vi "Configure Digitize Function.vi"(6 "Sample Rate (1E+6)":dbl=1000000.0, 7 "Manual Range (0)":dbl=1.0, 8 "error in (no error)":errorcluster, 9 "Count (1)":u32=1, 10 "Function":u16(ring) items=["Digitize Voltage", "Digitize Current"], 11 "VISA resource name":refnum<visa-resource-name>) -> (0 "error out":errorcluster, 3 "VISA resource name out":refnum<visa-resource-name>)   [LabVIEW 2025, in "Keithley DMM7510.lvlib"]
doc: "This VI selects which type of digitize function is active."
uses:
  Keithley DMM7510.lvlib
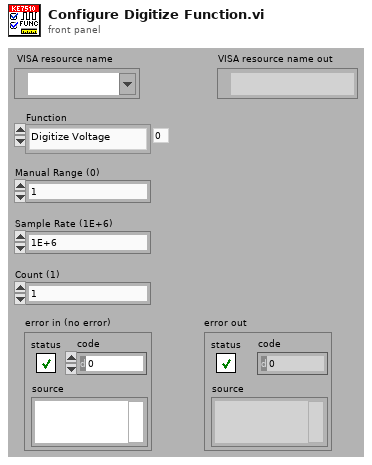
[diagram p1: front panel]
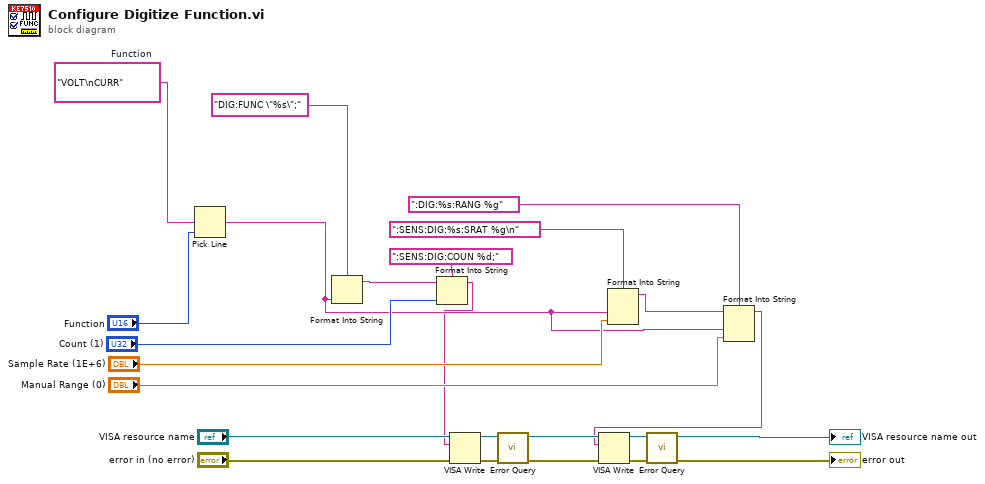
[diagram p0: block diagram]
diagram:
  w19 = "VOLT\nCURR"  # Function
  n1 = Pick Line(multi-line string=w19, line index="Function") -> (output string=w12:string)  [unwired: 1 out]
  n2 = Format Into String(format string="DIG:FUNC \"%s\";", w12) -> (resulting string=w10:string)  [unwired: 2 in, 1 out]
  n3 = Format Into String(format string=":SENS:DIG:COUN %d;", initial string=w10, "Count (1)") -> (resulting string=w9:string)  [unwired: 1 in, 1 out]
  n4 = VISA Write(VISA resource name="VISA resource name", write buffer=w9, error in (no error)="error in (no error)") -> (VISA resource name out=w22:refnum<visa-resource-name>, error out=w21:errorcluster)  [unwired: 1 out]
  n5 = call "Error Query.vi"("error in (no error)"=w21, "VISA resource name"=w22) -> ("error out"=w5:errorcluster, "VISA resource name out"=w6:refnum<visa-resource-name>)  [unwired: 8 out]
  n6 = Format Into String(format string=":SENS:DIG:%s:SRAT %g\n", w12, "Sample Rate (1E+6)") -> (resulting string=w2:string)  [unwired: 2 in, 1 out]
  n7 = Format Into String(format string=":DIG:%s:RANG %g", initial string=w2, w12, "Manual Range (0)") -> (resulting string=w1:string)  [unwired: 1 in, 1 out]
  n8 = VISA Write(VISA resource name=w6, write buffer=w1, error in (no error)=w5) -> (VISA resource name out=w8:refnum<visa-resource-name>, error out=w7:errorcluster)  [unwired: 1 out]
  n9 = call "Error Query.vi"("error in (no error)"=w7, "VISA resource name"=w8) -> ("error out"=→"error out":errorcluster, "VISA resource name out"=→"VISA resource name out":refnum<visa-resource-name>)  [unwired: 8 out]
